vi "Databse State Checker.vi"(8 "error in (no error)":errorcluster, 9 "connection information":path, 10 "System Number":string, 11 "Arduino in":refnum<visa-resource-name>="COM4") -> (0 "error out":errorcluster, 2 "Database Available?":bool, 3 "Arduino out":refnum<visa-resource-name>)   [LabVIEW 2024]
uses:
  <vilib>/addons/database/Connection.llb/DB Tools Open Connec (Path).vi
  <vilib>/addons/database/_DB Variant To Data/Database Variant To Data.xnode
  <vilib>/regexp/Match Regular Expression.xnode
  <vilib>/addons/database/NI_Database_API.lvlib
panel:
  out "Command Array":string[](array[string])
  out "Power":string[](array[string])
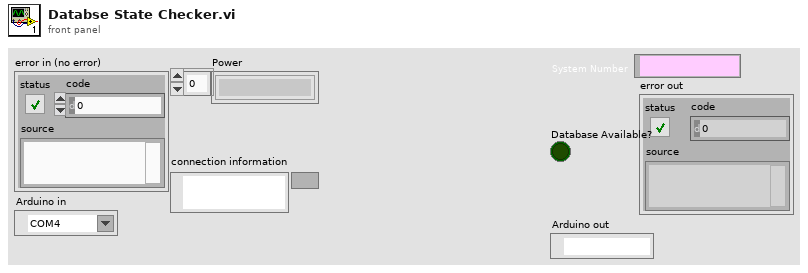
[diagram p1: front panel]
types:
  T1 = typedef "NI_Database_API.lvlib/Conn ObjectReference.ctl" = refnum<k1>
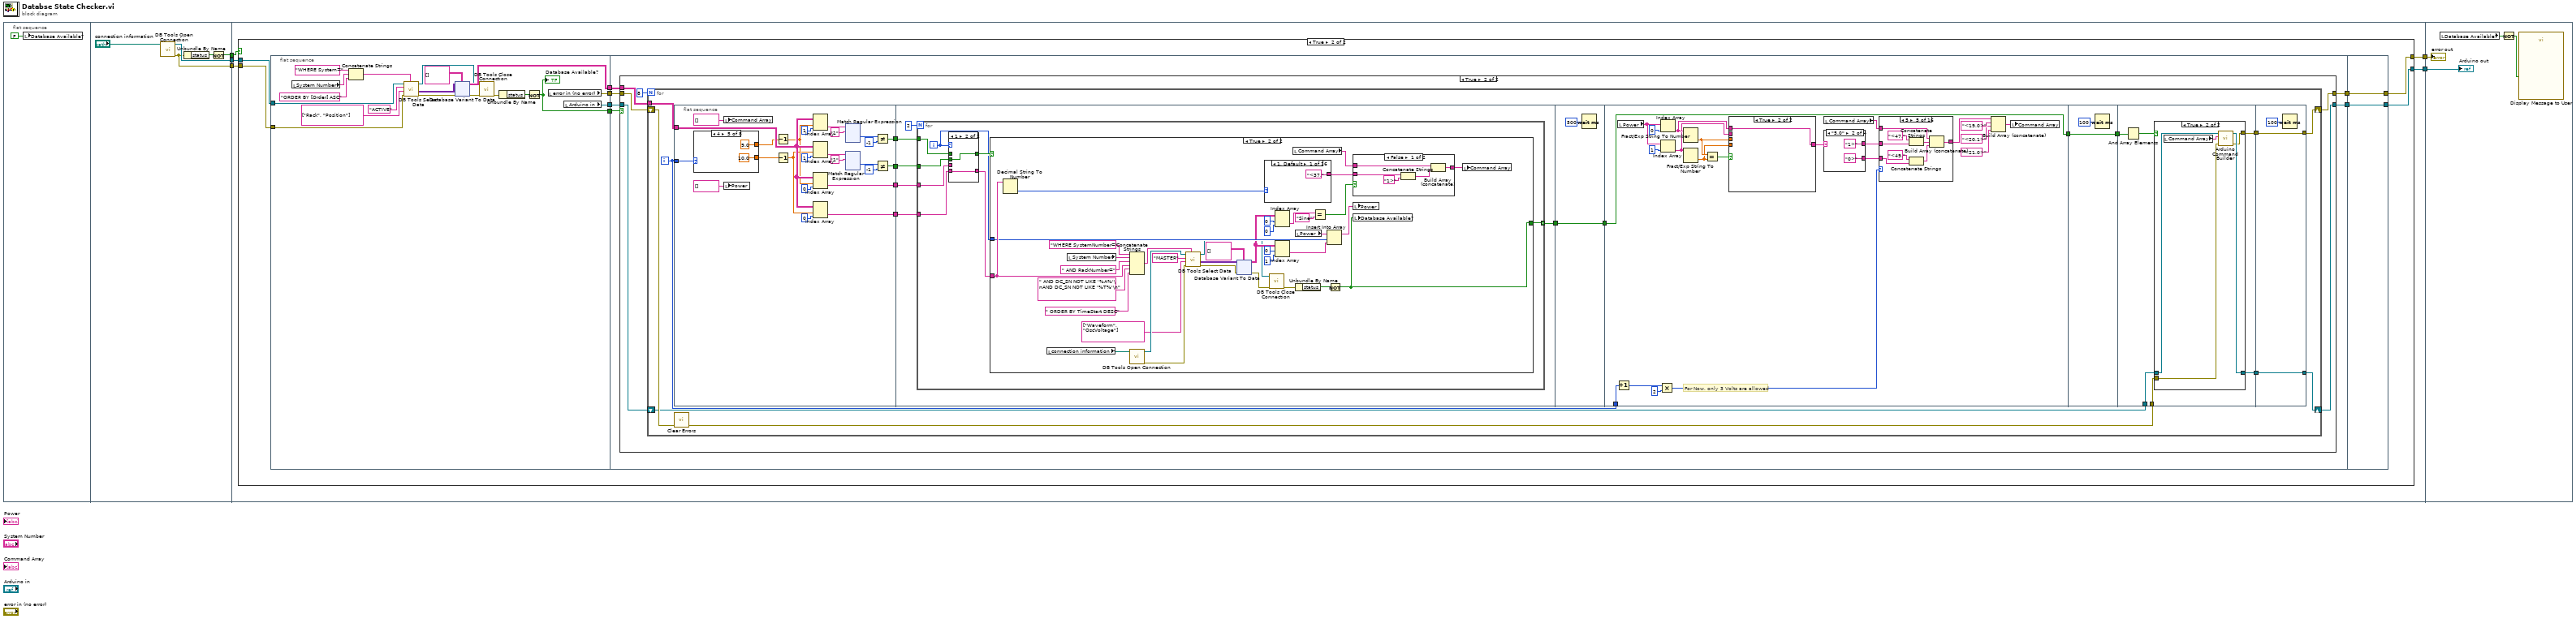
[diagram p0: block diagram]
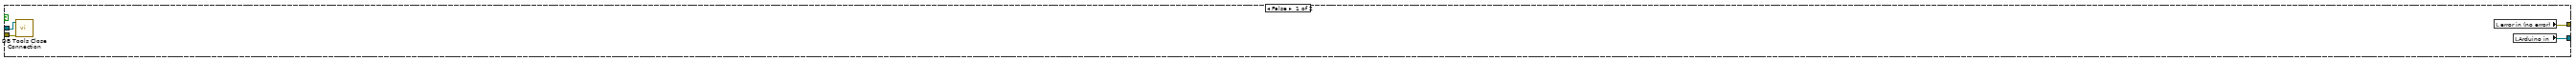
[diagram p2: hidden frame]
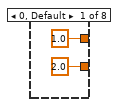
[diagram p4: hidden frame]
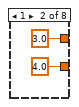
[diagram p5: hidden frame]
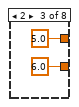
[diagram p6: hidden frame]
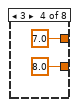
[diagram p7: hidden frame]
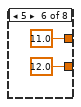
[diagram p8: hidden frame]
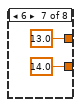
[diagram p9: hidden frame]
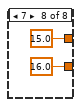
[diagram p10: hidden frame]
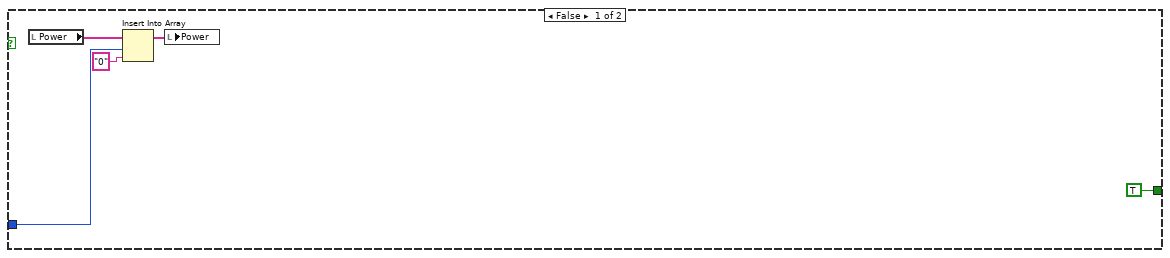
[diagram p12: hidden frame]
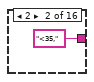
[diagram p13: hidden frame]
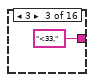
[diagram p14: hidden frame]
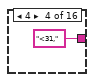
[diagram p15: hidden frame]
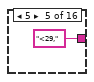
[diagram p16: hidden frame]
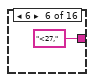
[diagram p17: hidden frame]
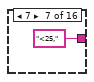
[diagram p18: hidden frame]
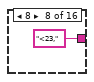
[diagram p19: hidden frame]
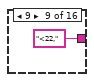
[diagram p20: hidden frame]
diagram:
  n1 = flat-sequence {
    tunnel: [w10] -> w3
    tunnel: [w7] -> w2
    tunnel: [w8] -> w1
    tunnel: [w15] -> w5
    tunnel: [w14] -> w4
    tunnel: w3 -> [w16]
    tunnel: w2 -> [w13]
    tunnel: w1 -> [w12]
    tunnel: w5 -> [w719]
    tunnel: w4 -> [w718]
    frame #0 {
      n2 = local write "Database Available?"(FALSE ("Database Available?")) -> ()
    }
    frame #1 {
      n3 = call-poly <vilib>:"DB Tools Open Connection.vi"("connection information"="connection information") -> ("error out"=w7:errorcluster, "connection reference"=w8:T1)  [unwired: 7 in]
      n4 = Unbundle By Name(w7) -> ("status"=w11:bool)
      n5 = Not(x=w11) -> (.not. x?=w10:bool)
    }
    frame #2 {
      n6 = case shown="True" w16 {
        tunnel: [w19 w26] -> w15
        tunnel: [w20 w25] -> w14
        tunnel: w13 -> [w17 w22]
        tunnel: w12 -> [w18 w21]
        frame False {
          n7 = call <vilib>:"DB Tools Close Connection.vi"("error in (no error)"=w17, "connection reference"=w18) -> ()  [unwired: 5 in, 1 out]
          n8 = local read "error in (no error)"() -> (w20:errorcluster)
          n9 = local read "Arduino in"() -> (w19:refnum<visa-resource-name>)
        }
        frame True {
          n10 = flat-sequence {
            tunnel: [w35] -> w30
            tunnel: [w49] -> w29
            tunnel: [w48] -> w28
            tunnel: [w46] -> w27
            tunnel: w22 -> [w39]
            tunnel: w21 -> [w38]
            tunnel: w30 -> [w97]
            tunnel: w29 -> [w96]
            tunnel: w28 -> [w94]
            tunnel: w27 -> [w95]
            tunnel: [w99] -> w24
            tunnel: [w98] -> w23
            tunnel: [w714] -> w25
            tunnel: [w715] -> w26
            tunnel: w24 -> [w715]
            tunnel: w23 -> [w714]
            frame #0 {
              n11 = local read "System Number"() -> (w45:string)
              n12 = Concatenate Strings("WHERE System=" ("SQL Query"), w45, "ORDER BY [Order] ASC" ("string")) -> (w37:string)
              n13 = call <vilib>:"DB Tools Select Data.vi"("condition"=w37, "error in (no error)"=w39, "columns"=string[] ["Rack", "Position"], "table"="ACTIVE", "connection reference"=w38) -> ("error out"=w36:errorcluster, "data"=w41:variant[][], "connection reference out"=w31:T1)  [unwired: 1 in]
              n14 = xnode "Database Variant To Data"("database variant"=w41, "error in (no error)"=w36, "type"=string[][] [] ("table")) -> ("data"=w35:string[][], "error out"=w33:errorcluster)
              n15 = call <vilib>:"DB Tools Close Connection.vi"("error in (no error)"=w33, "connection reference"=w31) -> ("error out"=w32:errorcluster)  [unwired: 5 in]
              n16 = Unbundle By Name(w32) -> ("status"=w47:bool)
              n17 = Not(x=w47) -> (.not. x?=w46:bool)
              "Database Available?" <- w46
              n18 = local read "error in (no error)"() -> (w48:errorcluster)
              n19 = local read "Arduino in"() -> (w49:refnum<visa-resource-name>)
            }
            frame #1 {
              n20 = case shown="True" w95 {
                tunnel: [w101 w107] -> w99
                tunnel: [w100 w106] -> w98
                tunnel: w96 -> [w101 w105]
                tunnel: w94 -> [w100 w104]
                tunnel: w97 -> [_ w103]
                frame False {
                }
                frame True {
                  n21 = for {
                    N: 8 -> [_]
                    tunnel: w103 -> [w124]
                    shift-right: [w121] -> w107
                    shift-left: w105 -> [w112]
                    shift-right: [w120] -> w106
                    shift-left: w104 -> [w119]
                    i -> [w116]
                    n22 = flat-sequence {
                      tunnel: w124 -> [w138]
                      tunnel: w116 -> [w137]
                      tunnel: [w145] -> w123
                      tunnel: [w144] -> w122
                      tunnel: [w128] -> w118
                      tunnel: [w127] -> w117
                      tunnel: w123 -> [w404]
                      tunnel: w122 -> [w403]
                      tunnel: w118 -> [w401]
                      tunnel: w117 -> [w400]
                      tunnel: [w399] -> w110
                      tunnel: [w528] -> w111
                      tunnel: w110 -> [w528]
                      tunnel: w116 -> [w544]
                      tunnel: w111 -> [w535]
                      tunnel: [w535] -> w108
                      tunnel: [w696] -> w109
                      tunnel: w108 -> [w696]
                      tunnel: [w701] -> w115
                      tunnel: [w700] -> w114
                      tunnel: w113 -> [w703]
                      tunnel: w112 -> [w702]
                      tunnel: w109 -> [w699]
                      tunnel: [w712] -> w120
                      tunnel: [w713] -> w121
                      tunnel: w114 -> [w712]
                      tunnel: w115 -> [w713]
                      frame #0 {
                        n23 = case shown="4" w137 {
                          tunnel: [2.0 4.0 6.0 8.0 10.0 12.0 14.0 16.0] -> w131
                          tunnel: [1.0 3.0 5.0 7.0 9.0 11.0 13.0 15.0] -> w132
                          frame 0, Default {
                          }
                          frame 1 {
                          }
                          frame 2 {
                          }
                          frame 3 {
                          }
                          frame 4 {
                          }
                          frame 5 {
                          }
                          frame 6 {
                          }
                          frame 7 {
                          }
                        }
                        n24 = local write "Command Array"(string[] [] ("array")) -> ()
                        n25 = local write "Power"(string[] [] ("array")) -> ()
                        n26 = Decrement(x=w132) -> (x-1=w130:dbl)
                        n27 = Decrement(x=w131) -> (x-1=w129:dbl)
                        n28 = Index Array(array=w138, index (row)=w130, index (col)=1 ("index")) -> (element=w143:string)
                        n29 = Index Array(array=w138, index (row)=w129, index (col)=1 ("index")) -> (element=w139:string)
                        n30 = Index Array(array=w138, index (row)=w130, index (col)=0 ("index")) -> (element=w145:string)
                        n31 = Index Array(array=w138, index (row)=w129, index (col)=0 ("index")) -> (element=w127:string)
                        n32 = xnode "Match Regular Expression"("input string"=w143, "regular expression"="1") -> ("offset past match"=w147:i32)  [unwired: 4 in, 4 out]
                        n33 = xnode "Match Regular Expression"("input string"=w139, "regular expression"="1") -> ("offset past match"=w141:i32)  [unwired: 4 in, 4 out]
                        n34 = Not Equal?(x=w147, y=-1) -> (x != y?=w144:bool)
                        n35 = Not Equal?(x=w141, y=-1) -> (x != y?=w128:bool)
                      }
                      frame #1 {
                        n36 = for {
                          N: 2 -> [_]
                          tunnel: w404 -> [w409]
                          tunnel: w403 -> [w410]
                          tunnel: w401 -> [w411]
                          tunnel: w400 -> [w412]
                          tunnel: [w405] -> w399 mode=indexing
                          i -> [w406]
                          n37 = case shown="1" w406 {
                            tunnel: w412 -> [_ w416]
                            tunnel: [w413 w416] -> w408
                            tunnel: w411 -> [_ w415]
                            tunnel: [w414 w415] -> w407
                            tunnel: w410 -> [w414 _]
                            tunnel: w409 -> [w413 _]
                            frame 0, Default {
                            }
                            frame 1 {
                            }
                          }
                          n38 = case shown="True" w407 {
                            tunnel: w408 -> [_ w457]
                            tunnel: w406 -> [w418 w456]
                            tunnel: [TRUE w424] -> w405
                            frame False {
                              n39 = local read "Power"() -> (w421:string[])
                              n40 = Insert Into Array(array=w421, index=w418, new element="0" ("new element/subarray")) -> (w420:string[])
                              n41 = local write "Power"(w420) -> ()
                            }
                            frame True {
                              n42 = Decimal String To Number(string=w457) -> (number=w440:i32)  [unwired: 2 in, 1 out]
                              n43 = local read "connection information"() -> (w422:path)
                              n44 = local read "System Number"() -> (w453:string)
                              n45 = Concatenate Strings("WHERE SystemNumber=" ("string"), w453, " AND RackNumber=", w457, " AND DC_SN NOT LIKE '%A%'\nAND DC_SN NOT LIKE '%T%'\n" ("string"), " ORDER BY TimeStart DESC" ("string")) -> (w431:string)
                              n46 = call-poly <vilib>:"DB Tools Open Connection.vi"("connection information"=w422) -> ("error out"=w428:errorcluster, "connection reference"=w429:T1)  [unwired: 7 in]
                              n47 = call <vilib>:"DB Tools Select Data.vi"("condition"=w431, "error in (no error)"=w428, "columns"=string[] ["Waveform", "OscVoltage"], "table"="MASTER", "connection reference"=w429) -> ("error out"=w432:errorcluster, "data"=w434:variant[][], "connection reference out"=w426:T1)  [unwired: 1 in]
                              n48 = xnode "Database Variant To Data"("database variant"=w434, "error in (no error)"=w432, "type"=string[][] [] ("table")) -> ("data"=w430:string[][], "error out"=w425:errorcluster)
                              n49 = case shown="1, Default" w440 {
                                tunnel: ["<37," ("y") "<35," ("y") "<33," ("y") "<31," ("y") "<29," ("y") "<27," ("y") "<25," ("y") "<23," ("y") "<22," ("y") "<24," ("y") "<26," ("y") "<28," ("y") "<30," ("y") "<32," ("y") "<34," ("y") "<36," ("y")] -> w437
                                frame 1, Default {
                                }
                                frame 2 {
                                }
                                frame 3 {
                                }
                                frame 4 {
                                }
                                frame 5 {
                                }
                                frame 6 {
                                }
                                frame 7 {
                                }
                                frame 8 {
                                }
                                frame 9 {
                                }
                                frame 10 {
                                }
                                frame 11 {
                                }
                                frame 12 {
                                }
                                frame 13 {
                                }
                                frame 14 {
                                }
                                frame 15 {
                                }
                                frame 16 {
                                }
                              }
                              n50 = call <vilib>:"DB Tools Close Connection.vi"("error in (no error)"=w425, "connection reference"=w426) -> ("error out"=w427:errorcluster)  [unwired: 5 in]
                              n51 = Index Array(array=w430, index (row)=0 ("index"), index (col)=0 ("disabled index (col)")) -> (element=w448:string)
                              n52 = Index Array(array=w430, index (row)=0, index (col)=1 ("disabled index (col)")) -> (element=w445:string)
                              n53 = local read "Command Array"() -> (w438:string[])
                              n54 = local read "Power"() -> (w443:string[])
                              n55 = Unbundle By Name(w427) -> ("status"=w436:bool)
                              n56 = Equal?(x=w448, y="Sine") -> (x = y?=w446:bool)
                              n57 = Insert Into Array(array=w443, index=w456, new element=w445) -> (w444:string[])
                              n58 = Not(x=w436) -> (.not. x?=w424:bool)
                              n59 = case shown="False" w446 {
                                tunnel: [w521 w527] -> w439
                                tunnel: w438 -> [w522 w526]
                                tunnel: w437 -> [w518 w523]
                                frame False {
                                n60 = Concatenate Strings(w518, "1>" ("y")) -> (w520:string)
                                n61 = Build Array (concatenate)(w522, w520) -> (w521:string[])
                                }
                                frame True {
                                n62 = Concatenate Strings(w523, "0>" ("y")) -> (w525:string)
                                n63 = Build Array (concatenate)(w526, w525) -> (w527:string[])
                                }
                              }
                              n64 = local write "Power"(w444) -> ()
                              n65 = local write "Database Available?"(w424) -> ()
                              n66 = local write "Command Array"(w439) -> ()
                            }
                          }
                        }
                      }
                      frame #2 {
                        n67 = Wait (ms)(milliseconds to wait=u32 500) -> ()  [unwired: 1 out]
                      }
                      frame #3 {
                        # "For Now, only 3 Volts are allowed"
                        n68 = Increment(x=w544) -> (x+1=w543:i32)
                        n69 = local read "Power"() -> (w549:string[])
                        n70 = Multiply(x=w543, y=2) -> (x*y=w541:i32)
                        n71 = Index Array(array=w549, index=0) -> (element=w547:string)
                        n72 = Index Array(array=w549, index=1) -> (element=w546:string)
                        n73 = Fract/Exp String To Number(string=w547) -> (number=w540:dbl)  [unwired: 3 in, 1 out]
                        n74 = Fract/Exp String To Number(string=w546) -> (number=w539:dbl)  [unwired: 3 in, 1 out]
                        n75 = Equal?(x=w540, y=w539) -> (x = y?=w548:bool)
                        n76 = case shown="True" w548 {
                          tunnel: w547 -> [w561 w567]
                          tunnel: w546 -> [w560 _]
                          tunnel: [w559 w567] -> w545
                          tunnel: w540 -> [w563 _]
                          tunnel: w539 -> [w564 _]
                          frame False {
                            n77 = Greater?(x=w563, y=w564) -> (0:w562:bool)
                            n78 = case shown="True" w562 {
                              tunnel: w561 -> [_ w566]
                              tunnel: w560 -> [w565 _]
                              tunnel: [w565 w566] -> w559
                              frame False {
                              }
                              frame True {
                              }
                            }
                          }
                          frame True {
                          }
                        }
                        n79 = case shown="\"5.0\"" w545 {
                          tunnel: [w552 "1>" "0>" "0>"] -> w538
                          tunnel: [w552 "0>" "1>" "1>"] -> w537
                          frame "0", Default {
                            w552 = "0>"
                          }
                          frame "5.0" {
                          }
                          frame "12.0" {
                          }
                          frame "3.3" {
                          }
                        }
                        n80 = local read "Command Array"() -> (w536:string[])
                        n81 = case shown="5" w541 {
                          tunnel: w538 -> [w574 w582 w590 w598 w606 w614 w622 w630 w638 w646 w654 w662 w670 w678 w686 w694]
                          tunnel: w537 -> [w575 w583 w591 w599 w607 w615 w623 w631 w639 w647 w655 w663 w671 w679 w687 w695]
                          tunnel: w536 -> [w569 w577 w585 w593 w601 w609 w617 w625 w633 w641 w649 w657 w665 w673 w681 w689]
                          tunnel: [w568 w576 w584 w592 w600 w608 w616 w624 w632 w640 w648 w656 w664 w672 w680 w688] -> w534
                          frame 1, Default {
                            n82 = Concatenate Strings("<39,", w574) -> (w571:string)
                            n83 = Concatenate Strings("<41,", w575) -> (w570:string)
                            n84 = Build Array (concatenate)(w569, w571, w570) -> (w568:string[])
                          }
                          frame 2 {
                            n85 = Concatenate Strings("<39,", w582) -> (w579:string)
                            n86 = Concatenate Strings("<41,", w583) -> (w578:string)
                            n87 = Build Array (concatenate)(w577, w579, w578) -> (w576:string[])
                          }
                          frame 3 {
                            n88 = Concatenate Strings("<43,", w590) -> (w587:string)
                            n89 = Concatenate Strings("<45,", w591) -> (w586:string)
                            n90 = Build Array (concatenate)(w585, w587, w586) -> (w584:string[])
                          }
                          frame 4 {
                            n91 = Concatenate Strings("<43,", w598) -> (w595:string)
                            n92 = Concatenate Strings("<45,", w599) -> (w594:string)
                            n93 = Build Array (concatenate)(w593, w595, w594) -> (w592:string[])
                          }
                          frame 5 {
                            n94 = Concatenate Strings("<47,", w606) -> (w603:string)
                            n95 = Concatenate Strings("<49,", w607) -> (w602:string)
                            n96 = Build Array (concatenate)(w601, w603, w602) -> (w600:string[])
                          }
                          frame 6 {
                            n97 = Concatenate Strings("<47,", w614) -> (w611:string)
                            n98 = Concatenate Strings("<49,", w615) -> (w610:string)
                            n99 = Build Array (concatenate)(w609, w611, w610) -> (w608:string[])
                          }
                          frame 7 {
                            n100 = Concatenate Strings("<51,", w622) -> (w619:string)
                            n101 = Concatenate Strings("<53,", w623) -> (w618:string)
                            n102 = Build Array (concatenate)(w617, w619, w618) -> (w616:string[])
                          }
                          frame 8 {
                            n103 = Concatenate Strings("<51,", w630) -> (w627:string)
                            n104 = Concatenate Strings("<53,", w631) -> (w626:string)
                            n105 = Build Array (concatenate)(w625, w627, w626) -> (w624:string[])
                          }
                          frame 9 {
                            n106 = Concatenate Strings("<52,", w638) -> (w635:string)
                            n107 = Concatenate Strings("<50,", w639) -> (w634:string)
                            n108 = Build Array (concatenate)(w633, w635, w634) -> (w632:string[])
                          }
                          frame 10 {
                            n109 = Concatenate Strings("<52,", w646) -> (w643:string)
                            n110 = Concatenate Strings("<50,", w647) -> (w642:string)
                            n111 = Build Array (concatenate)(w641, w643, w642) -> (w640:string[])
                          }
                          frame 11 {
                            n112 = Concatenate Strings("<48,", w654) -> (w651:string)
                            n113 = Concatenate Strings("<46,", w655) -> (w650:string)
                            n114 = Build Array (concatenate)(w649, w651, w650) -> (w648:string[])
                          }
                          frame 12 {
                            n115 = Concatenate Strings("<48,", w662) -> (w659:string)
                            n116 = Concatenate Strings("<46,", w663) -> (w658:string)
                            n117 = Build Array (concatenate)(w657, w659, w658) -> (w656:string[])
                          }
                          frame 13 {
                            n118 = Concatenate Strings("<44,", w670) -> (w667:string)
                            n119 = Concatenate Strings("<42,", w671) -> (w666:string)
                            n120 = Build Array (concatenate)(w665, w667, w666) -> (w664:string[])
                          }
                          frame 14 {
                            n121 = Concatenate Strings("<44,", w678) -> (w675:string)
                            n122 = Concatenate Strings("<42,", w679) -> (w674:string)
                            n123 = Build Array (concatenate)(w673, w675, w674) -> (w672:string[])
                          }
                          frame 15 {
                            n124 = Concatenate Strings("<40,", w686) -> (w683:string)
                            n125 = Concatenate Strings("<38,", w687) -> (w682:string)
                            n126 = Build Array (concatenate)(w681, w683, w682) -> (w680:string[])
                          }
                          frame 16 {
                            n127 = Concatenate Strings("<40,", w694) -> (w691:string)
                            n128 = Concatenate Strings("<38,", w695) -> (w690:string)
                            n129 = Build Array (concatenate)(w689, w691, w690) -> (w688:string[])
                          }
                        }
                        n130 = Build Array (concatenate)(w534, "<19,0>" ("y"), "<20,1>" ("y"), "<21,0>" ("y")) -> (w530:string[])
                        n131 = local write "Command Array"(w530) -> ()
                      }
                      frame #4 {
                        n132 = Wait (ms)(milliseconds to wait=u32 100) -> ()  [unwired: 1 out]
                      }
                      frame #5 {
                        n133 = And Array Elements(Boolean array=w699) -> (logical AND=w698:bool)
                        n134 = case shown="True" w698 {
                          tunnel: w703 -> [w704 w710]
                          tunnel: w702 -> [w705 w709]
                          tunnel: [w705 w708] -> w701
                          tunnel: [w704 w707] -> w700
                          frame False {
                          }
                          frame True {
                            n135 = local read "Command Array"() -> (w706:string[])
                            n136 = call "Arduino Command Builder.vi"("error in"=w710, "Commands"=w706, "Arduino in"=w709) -> ("error out"=w707:errorcluster, "Arduino out"=w708:refnum<visa-resource-name>)  [unwired: 7 in]
                          }
                        }
                      }
                      frame #6 {
                        n137 = Wait (ms)(milliseconds to wait=u32 100) -> ()  [unwired: 1 out]
                      }
                    }
                    n138 = call <vilib>:"Clear Errors.vi"("error in (no error)"=w119) -> ("error out"=w113:errorcluster)  [unwired: 5 in, 1 out]
                  }
                }
              }
            }
            frame #2 {
            }
          }
        }
      }
    }
    frame #3 {
      n139 = local read "Database Available?"() -> (w717:bool)
      n140 = Not(x=w717) -> (.not. x?=w716:bool)
      n141 = call "Display Message to User"("Enable"=w716) -> ()  [unwired: 9 in, 2 out]
      "error out" <- w718
      "Arduino out" <- w719
    }
  }
